vi "Calc P4.vi"(9 "Bottom":T1={"Position"={"x"=0.0, "y"=0.0, "z"=0.0}, "UV"={"u"=0.0, "v"=0.0}, "Colour"=12517256} {"UV"."v" min=0 max=1 step=0.1; "UV"."u" min=0 max=1 step=0.1}, 10 "Middle":T1={"Position"={"x"=0.0, "y"=0.0, "z"=0.0}, "UV"={"u"=0.0, "v"=0.0}, "Colour"=12517256} {"UV"."v" min=0 max=1 step=0.1; "UV"."u" min=0 max=1 step=0.1}, 11 "Top":T1={"Position"={"x"=0.0, "y"=0.0, "z"=0.0}, "UV"={"u"=0.0, "v"=0.0}, "Colour"=12517256} {"UV"."v" min=0 max=1 step=0.1; "UV"."u" min=0 max=1 step=0.1}) -> (3 "Point 4":T1={"Position"={"x"=0.0, "y"=0.0, "z"=0.0}, "UV"={"u"=0.0, "v"=0.0}, "Colour"=12517256} {"UV"."v" min=0 max=1 step=0.1; "UV"."u" min=0 max=1 step=0.1})   [LabVIEW 2020]
uses:
  Vertex.ctl
  Vector 3D.ctl
  UV.ctl
  Raster (FPGA).lvlib
panel:
  out "32bit integer":i32
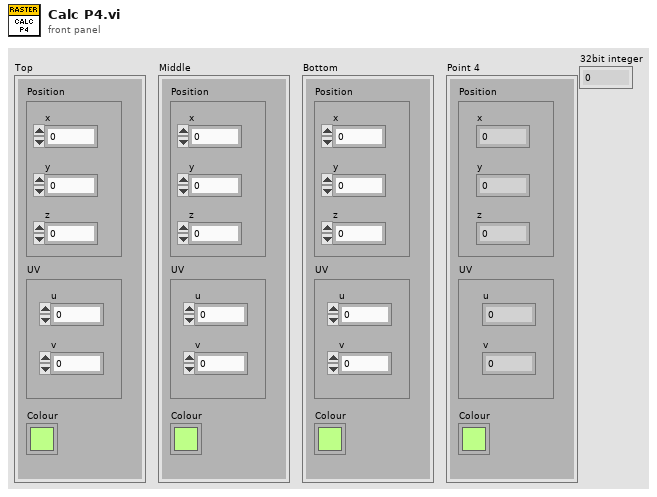
[diagram p1: front panel]
types:
  T1 = typedef "Raster (FPGA).lvlib/Vertex.ctl" = cluster{"Position":T2, "UV":T3, "Colour":u32}
  T2 = typedef "Raster (FPGA).lvlib/Vector 3D.ctl" = cluster{"x":sgl, "y":sgl, "z":sgl}
  T3 = typedef "Raster (FPGA).lvlib/UV.ctl" = cluster{"u":sgl, "v":sgl}
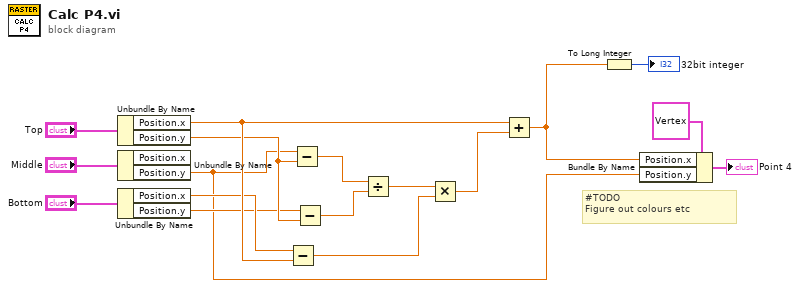
[diagram p0: block diagram]
diagram:
  # "#TODO\nFigure out colours etc"
  n1 = Unbundle By Name("Top") -> ("Position.x"=w8:sgl, "Position.y"=w5:sgl)
  n2 = Unbundle By Name("Middle") -> ("Position.y"=w3:sgl)  [unwired: 1 out]
  n3 = Unbundle By Name("Bottom") -> ("Position.x"=w7:sgl, "Position.y"=w4:sgl)
  n4 = Subtract(x=w7, y=w8) -> (x-y=w11:sgl)
  n5 = Subtract(x=w3, y=w5) -> (x-y=w6:sgl)
  n6 = Subtract(x=w4, y=w5) -> (x-y=w9:sgl)
  n7 = Divide(x=w6, y=w9) -> (x/y=w10:sgl)
  n8 = Multiply(x=w10, y=w11) -> (x*y=w12:sgl)
  n9 = Add(x=w8, y=w12) -> (x+y=w2:sgl)
  n10 = To Long Integer(number=w2) -> (32bit integer=→"32bit integer":i32)
  n11 = Bundle By Name(cluster=T1 {"Position"={"x"=0.0, "y"=0.0, "z"=0.0}, "UV"={"u"=0.0, "v"=0.0}, "Colour"=12517256} ("Point 1"), "Position.x"=w2, "Position.y"=w3) -> (→"Point 4":T1)
